vi "maszyna pomiar wirtualny.vi"() -> ()   [LabVIEW 2021]
uses:
  controlmaszyna.ctl
  <vilib>/Utility/file.llb/Write Delimited Spreadsheet (string).vi
panel:
  in  "W彻cz":bool
  in  "Wyjœcie":bool
  out "XY Graph":cluster{"Czêstotliwosc":dbl[], dbl[]}(graph)
  out "V out / V in":dbl[](array[numeric])
  out "Czêstotliwosc":dbl[](array[numeric])
  out "V in":dbl[](array[numeric])
  out "V out":dbl[](array[numeric])
  in  "Zapisz":bool
  in  "Zatrzymaj":bool
  in  "Rozpocznij":bool
  in  "Y LIN/LOG":bool
  in  "X LIN/LOG":bool
  in  "Amplituda":dbl
  in  "F min":dbl
  in  "Ilosc probek":u32
  in  "F max":dbl
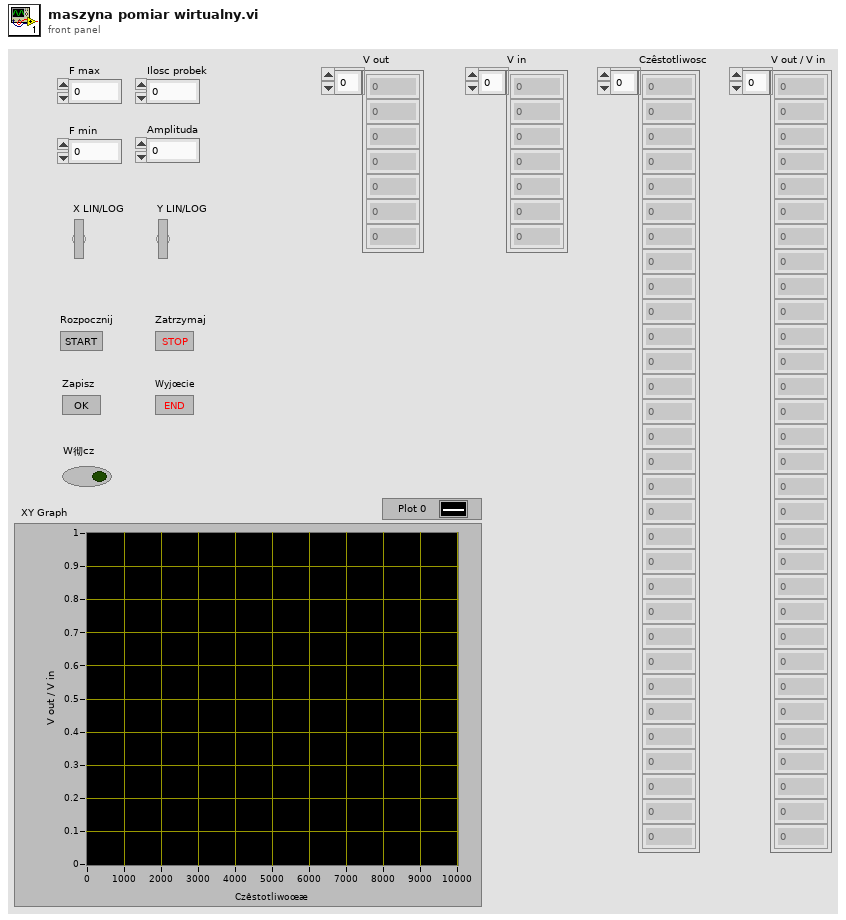
[diagram p1: front panel]
types:
  T1 = typedef "controlmaszyna.ctl" = enum16{"init", "praca", "pomiar", "wykres", "zapis", "stop", "koniec"}
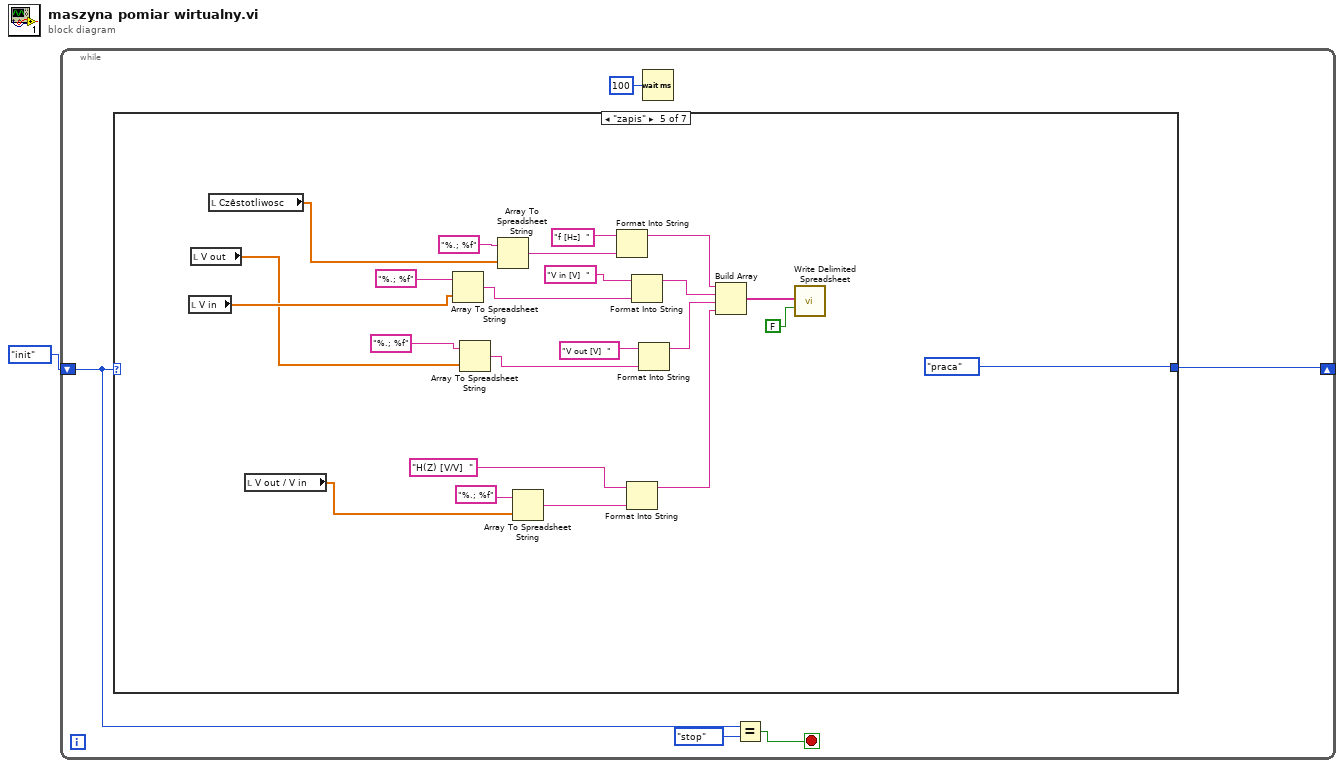
[diagram p0: block diagram]
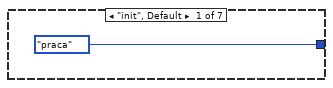
[diagram p2: hidden frame]
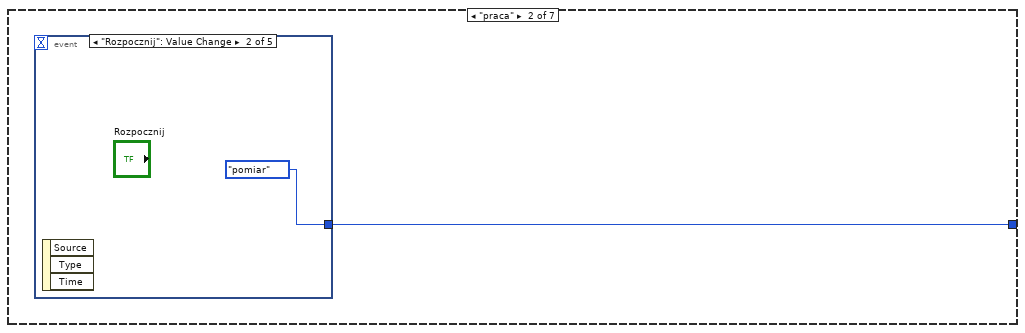
[diagram p3: hidden frame]
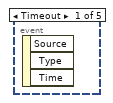
[diagram p4: hidden frame]
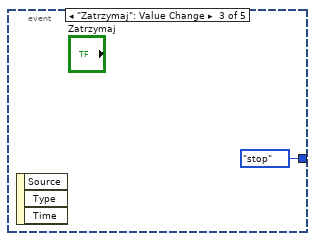
[diagram p5: hidden frame]
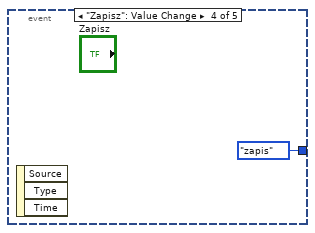
[diagram p6: hidden frame]
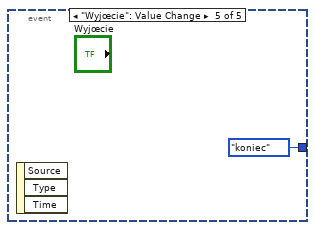
[diagram p7: hidden frame]
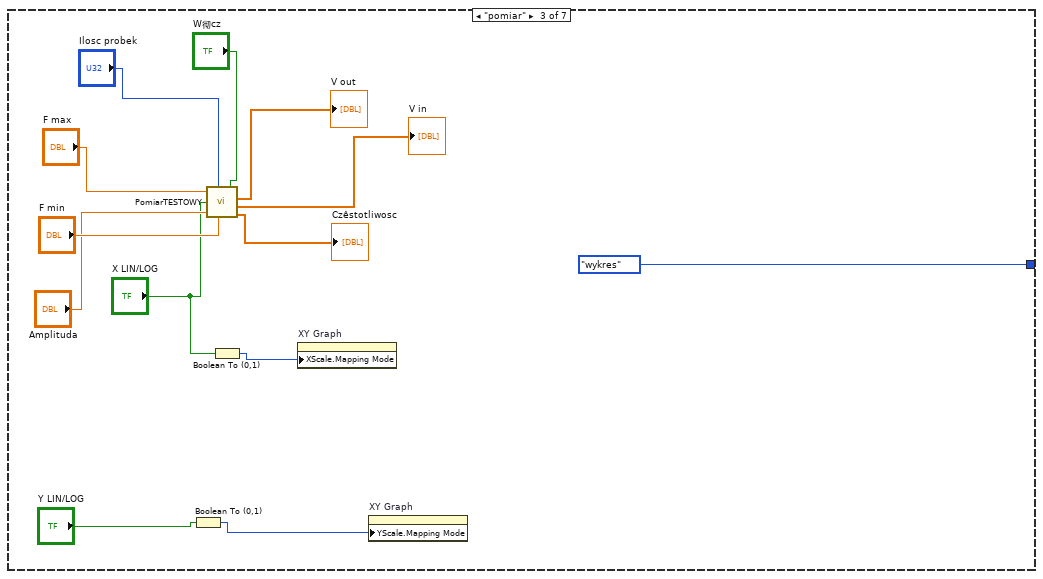
[diagram p8: hidden frame]
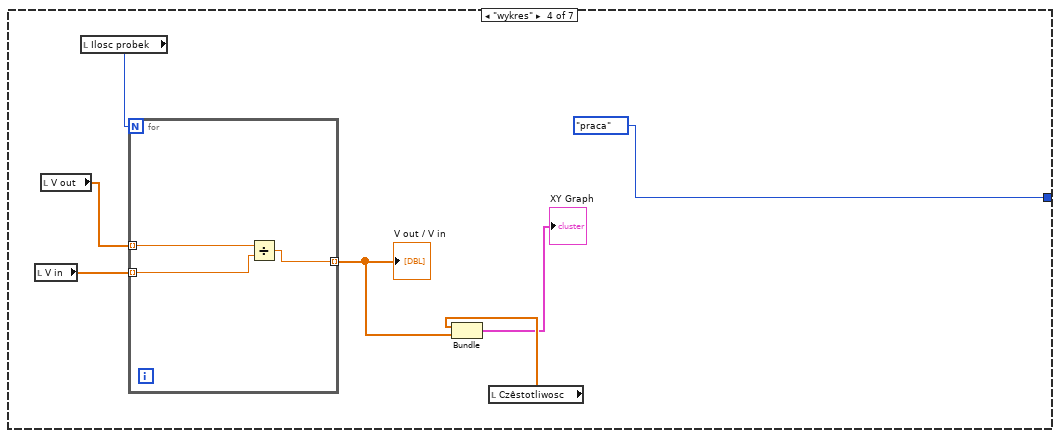
[diagram p9: hidden frame]
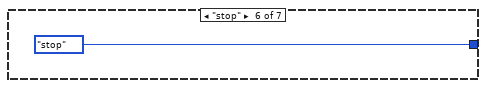
[diagram p10: hidden frame]
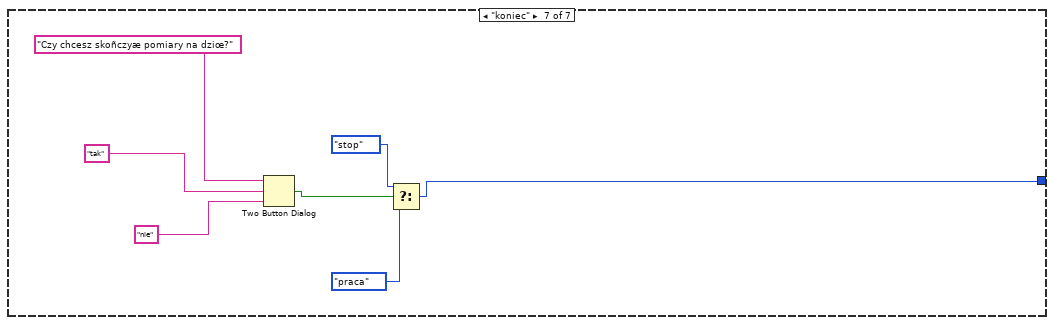
[diagram p11: hidden frame]
diagram:
  n1 = while {
    shift-right: [w6] -> _
    shift-left: controlmaszyna."init" -> [w5]
    stop <- w3 stop-if-true
    n2 = case shown="\"zapis\"" w5 {
      tunnel: [controlmaszyna."praca" w8 controlmaszyna."wykres" controlmaszyna."praca" controlmaszyna."praca" controlmaszyna."stop" w60] -> w6
      frame "init", Default {
      }
      frame "praca" {
        n3 = event shown="[1] \"Rozpocznij\": Value Change" {
          selector: _ -> [_ _ _ _ _]
          dyn-events: _ -> [_ _ _ _ _]
          timeout: _ -> [_ _ _ _ _]
          tunnel: [_ controlmaszyna."pomiar" controlmaszyna."stop" controlmaszyna."zapis" controlmaszyna."koniec"] -> w8
          event Timeout {
            n4 = event-data() -> ()  [unwired: 1 in, 3 out]
          }
          event "Rozpocznij": Value Change {
            n5 = event-data() -> ()  [unwired: 1 in, 3 out]
          }
          event "Zatrzymaj": Value Change {
            n6 = event-data() -> ()  [unwired: 1 in, 3 out]
          }
          event "Zapisz": Value Change {
            n7 = event-data() -> ()  [unwired: 1 in, 3 out]
          }
          event "Wyjœcie": Value Change {
            n8 = event-data() -> ()  [unwired: 1 in, 3 out]
          }
        }
      }
      frame "pomiar" {
        n9 = Boolean To (0,1)(Boolean="Y LIN/LOG") -> (0, 1=w16:i16)
        n10 = call "PomiarTESTOWY.vi"("F max"="F max", "ilosc probek"="Ilosc probek", "Liniowy/Logarytmiczny"="X LIN/LOG", "Amplituda"="Amplituda", "F min"="F min", "WLACZ"="W彻cz") -> ("V out"=→"V out":dbl[], "V in"=→"V in":dbl[], "Czestotliwosc"=→"Czêstotliwosc":dbl[])
        n11 = Boolean To (0,1)(Boolean="X LIN/LOG") -> (0, 1=w14:i16)
        n12 = property on="XY Graph" class="XYGraph (strict)"("XScale.Mapping Mode"=w14) -> ()  [unwired: 2 in, 2 out]
        n13 = property on="XY Graph" class="XYGraph (strict)"("YScale.Mapping Mode"=w16) -> ()  [unwired: 2 in, 2 out]
      }
      frame "wykres" {
        n14 = local read "V in"() -> (w30:dbl[])
        n15 = local read "V out"() -> (w31:dbl[])
        n16 = local read "Ilosc probek"() -> (w32:u32)
        n17 = for {
          N: w32 -> [_]
          tunnel: w31 -> [w35] mode=indexing
          tunnel: w30 -> [w34] mode=indexing
          tunnel: [w33] -> w29 mode=indexing
          n18 = Divide(x=w35, y=w34) -> (x/y=w33:dbl)
        }
        "V out / V in" <- w29
        n19 = local read "Czêstotliwosc"() -> (w28:dbl[])
        n20 = Bundle("Czêstotliwosc"=w28, w29) -> (→"XY Graph":cluster{"Czêstotliwosc":dbl[], dbl[]})  [unwired: 1 in]
      }
      frame "zapis" {
        n21 = local read "V in"() -> (w39:dbl[])
        n22 = local read "V out"() -> (w38:dbl[])
        n23 = local read "Czêstotliwosc"() -> (w40:dbl[])
        n24 = local read "V out / V in"() -> (w37:dbl[])
        n25 = Array To Spreadsheet String(array=w39, 3:"%.; %f" ("format string")) -> (spreadsheet string=w48:string)  [unwired: 1 in]
        n26 = Array To Spreadsheet String(array=w38, 3:"%.; %f" ("format string")) -> (spreadsheet string=w50:string)  [unwired: 1 in]
        n27 = Array To Spreadsheet String(array=w40, 3:"%.; %f" ("format string")) -> (spreadsheet string=w44:string)  [unwired: 1 in]
        n28 = Array To Spreadsheet String(array=w37, 3:"%.; %f" ("format string")) -> (spreadsheet string=w46:string)  [unwired: 1 in]
        n29 = Format Into String(initial string="f [Hz]  " ("element"), w44) -> (resulting string=w54:string)  [unwired: 2 in, 1 out]
        n30 = Format Into String(initial string="H(Z) [V/V]  ", w46) -> (resulting string=w57:string)  [unwired: 2 in, 1 out]
        n31 = Format Into String(initial string="V in [V]  " ("element"), w48) -> (resulting string=w55:string)  [unwired: 2 in, 1 out]
        n32 = Format Into String(initial string="V out [V]  " ("element"), w50) -> (resulting string=w56:string)  [unwired: 2 in, 1 out]
        n33 = Build Array(w54, w55, w56, w57) -> (w41:string[])
        n34 = call-poly <vilib>:"Write Delimited Spreadsheet.vi"("1D data"=w41, "append to file? (new file:F)"=FALSE) -> ()  [unwired: 12 in, 2 out]
      }
      frame "stop" {
      }
      frame "koniec" {
        n35 = Two Button Dialog(message="Czy chcesz skoñczyæ pomiary na dziœ?", 1:"nie" ("F button name (\"Cancel\")"), 2:"tak" ("T button name (\"OK\")")) -> (T button?=w63:bool)
        n36 = Select(t=controlmaszyna."stop", s=w63, f=controlmaszyna."praca") -> (s? t:f=w60:T1)
      }
    }
    n37 = Wait (ms)(milliseconds to wait=u32 100) -> ()  [unwired: 1 out]
    n38 = Equal?(x=w5, y=controlmaszyna."stop") -> (x = y?=w3:bool)
  }
